vi "factorial(feedback).vi"() -> ()   [LabVIEW 2014]
panel:
  out "factorial":dbl format="%#_13g"
  in  "input":dbl format="%#_13g"
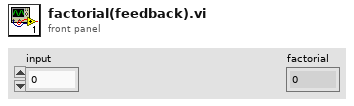
[diagram p1: front panel]
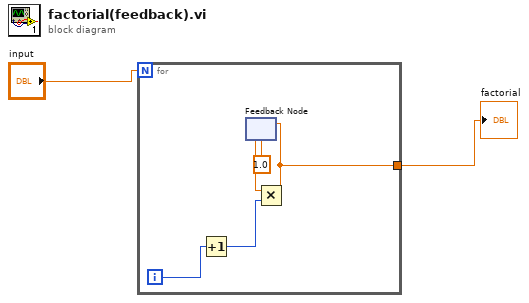
[diagram p0: block diagram]
diagram:
  n1 = for {
    N: "input" -> [_]
    tunnel: [w3] -> w1
    i -> [w7]
    n2 = Increment(x=w7) -> (x+1=w6:i32)
    n3 = feedback #1(1.0) -> (w5:dbl)
    n4 = Multiply(x=w5, y=w6) -> (x*y=w3:dbl)
    n5 = feedback-in #1(w3) -> ()
  }
  "factorial" <- w1
